vi "SubVI_Protocol_Calibration_Rev2.vi"(0 "TCP Network Connection in":refnum<k5>, 1 "ATAN scaler":dbl, 2 "Task":i32, 3 "Rest Period Length":i32, 4 "Current Level":dbl, 5 "error in (no error)":errorcluster, 6 "Total trial length":i32, 7 "Max Position":dbl, 8 "End of Imagine":i32, 9 "Target array":dbl[](array[numeric]), 10 "End of Fixate":i32, 11 "Arm Sampling Rate":u32, 17 "MidOut Proportion":dbl=0.55, 18 "Arm":string="right") -> (14 "TCP Network Connection out":refnum<k5>, 19 "error out":errorcluster)   [LabVIEW 2020]
uses:
  Global 1.vi
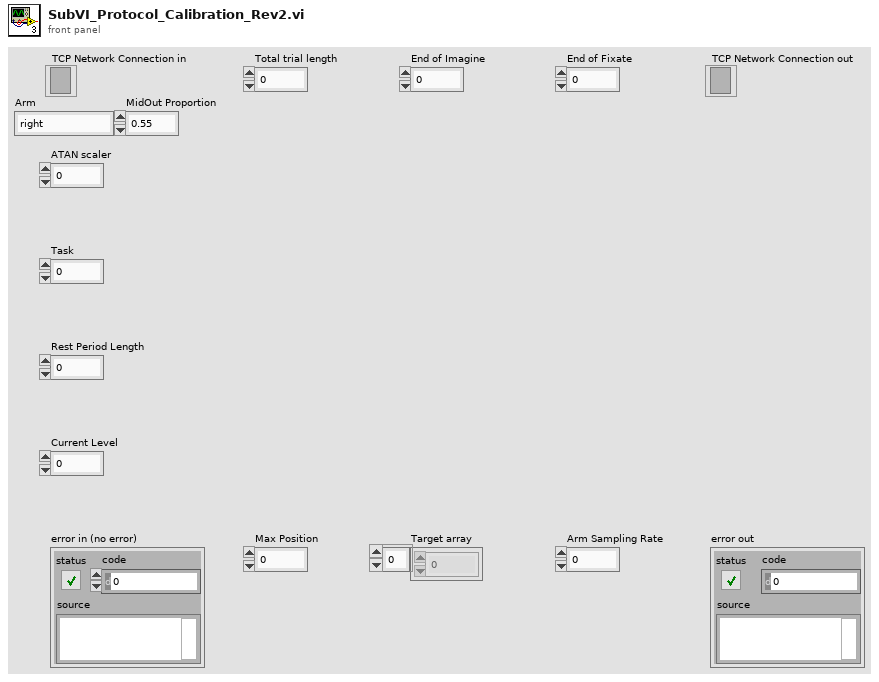
[diagram p1: front panel]
types:
  T1 = enum16{"Standard", "Buffered", "CRLF", "Immediate"}
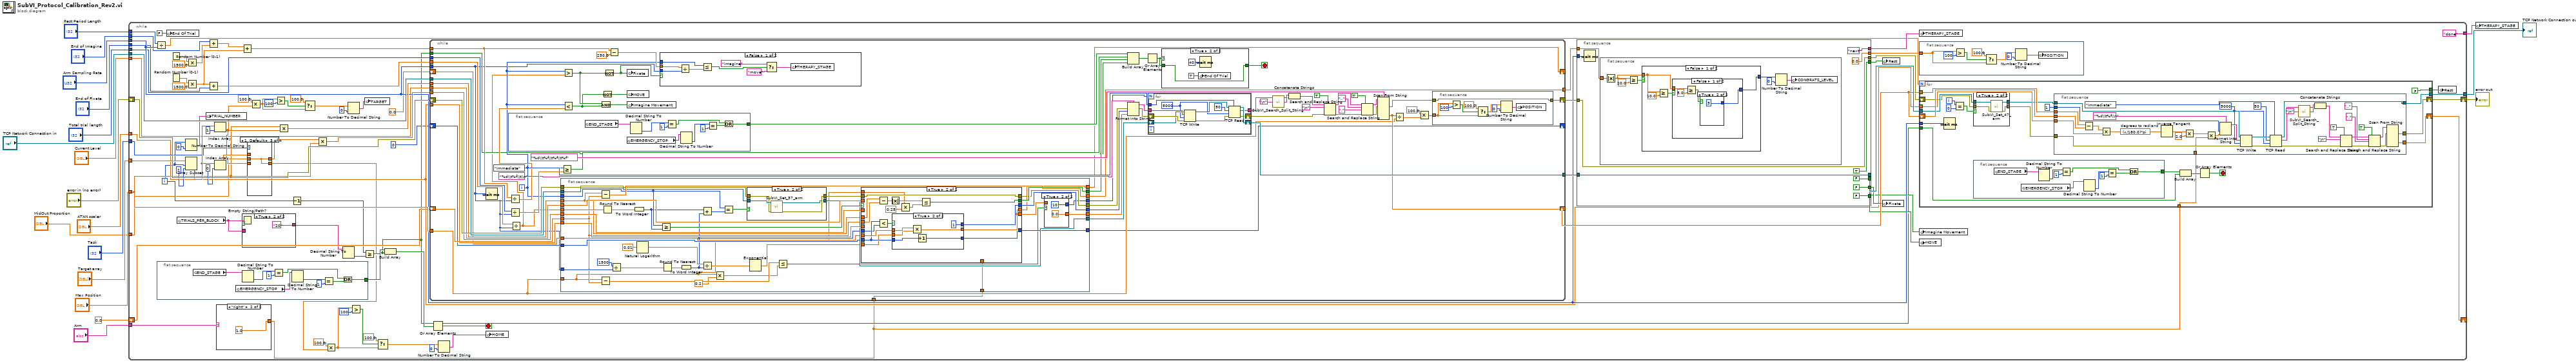
[diagram p0: block diagram]
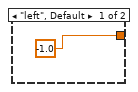
[diagram p2: hidden frame]
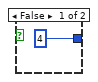
[diagram p5: hidden frame]
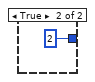
[diagram p6: hidden frame]
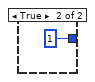
[diagram p7: hidden frame]
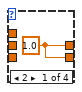
[diagram p8: hidden frame]
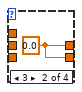
[diagram p9: hidden frame]
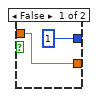
[diagram p13: hidden frame]
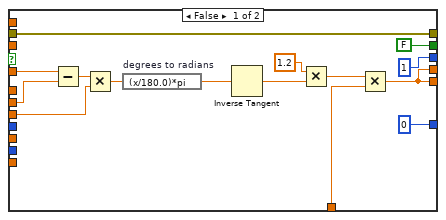
[diagram p14: hidden frame]
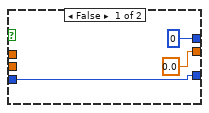
[diagram p15: hidden frame]
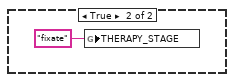
[diagram p16: hidden frame]
diagram:
  n1 = while {
    tunnel: "TCP Network Connection in" -> [w102]
    tunnel: [w64] -> w13
    shift-right: [w63] -> w14
    shift-left: "error in (no error)" -> [w101]
    tunnel: ["done" ("THERAPY_STAGE")] -> w17
    tunnel: "Arm Sampling Rate" -> [w61]
    tunnel: "Target array" -> [w99]
    tunnel: "Task" -> [w76]
    tunnel: "Max Position" -> [w71]
    tunnel: "Current Level" -> [w59]
    shift-right: [w65] -> _
    shift-left: 0.0 ("x") -> [w68]
    tunnel: "ATAN scaler" -> [w53]
    tunnel: "End of Fixate" -> [w41]
    tunnel: "End of Imagine" -> [w37]
    tunnel: "Total trial length" -> [w51]
    tunnel: "Rest Period Length" -> [w49]
    tunnel: "Arm" -> [w24]
    tunnel: "MidOut Proportion" -> [w21]
    i -> [w47]
    stop <- w29 stop-if-true
    n2 = Divide(x=w49, y=w61) -> (x/y=w60:dbl)
    n3 = flat-sequence {
      tunnel: [w105] -> w30
      frame #0 {
        n4 = global read "Global 1.vi" "END_STAGE"() -> (w113:string)
        n5 = global read "Global 1.vi" "EMERGENCY_STOP"() -> (w108:string)
        n6 = Decimal String To Number(string=w113) -> (number=w112:i32)  [unwired: 2 in, 1 out]
        n7 = Equal?(x=w112, y=1) -> (x = y?=w106:bool)
        n8 = Decimal String To Number(string=w108) -> (number=w110:i32)  [unwired: 2 in, 1 out]
        n9 = Equal?(x=w110, y=1) -> (x = y?=w107:bool)
        n10 = Or(x=w106, y=w107) -> (x .or. y?=w105:bool)
      }
    }
    n11 = global write "Global 1.vi" "End Of Trial"(FALSE ("End Of Trial")) -> ()
    n12 = Random Number (0-1)() -> (number: 0 to 1=w39:dbl)
    n13 = Random Number (0-1)() -> (number: 0 to 1=w43:dbl)
    n14 = global read "Global 1.vi" "TRIALS_PER_BLOCK"() -> (w45:string)
    n15 = Number To Decimal String(number=w47, width (-)=i16 0) -> (decimal integer string=w74:string)
    n16 = Array Subset(array=w99, index=w47, length=2) -> (w97:dbl[])
    n17 = Multiply(x=w39, y=1500.0) -> (x*y=w36:dbl)
    n18 = Multiply(x=w43, y=1500.0) -> (x*y=w34:dbl)
    n19 = global write "Global 1.vi" "TRIAL_NUMBER"(w74) -> ()
    n20 = Add(x=w37, y=w36) -> (x+y=w35:dbl)
    n21 = Add(x=w34, y=w41) -> (x+y=w40:dbl)
    n22 = Index Array(array=w97, index=1) -> (element=w79:dbl)
    n23 = Index Array(array=w97, index=0) -> (element=w94:dbl)
    n24 = case shown="\"right\"" w24 {
      tunnel: [-1.0 1.0] -> w25
      frame "left", Default {
      }
      frame "right" {
      }
    }
    n25 = Add(x=w35, y=w34) -> (x+y=w33:dbl)
    n26 = Empty String/Path?(string/path=w45) -> (empty?=w46:bool)
    n27 = case shown="True" w46 {
      tunnel: w45 -> [w114 _]
      tunnel: [w114 "20" ("TRIALS_PER_BLOCK")] -> w44
      frame False {
      }
      frame True {
      }
    }
    n28 = case shown="1, Default" w76 {
      tunnel: [w227 w228 w229 w231] -> w20
      tunnel: w94 -> [_ _ _ w231]
      tunnel: w79 -> [_ _ _ w230]
      tunnel: [w227 w228 w229 w230] -> w19
      tunnel: w21 -> [_ _ w229 _]
      frame 2 {
        w227 = 1.0
      }
      frame 3 {
        w228 = 0.0
      }
      frame 1, Default {
      }
      frame 0 {
      }
    }
    n29 = Multiply(x=100.0, y=w79) -> (x*y=w89:dbl)
    n30 = Greater?(x=w89, y=100) -> (0:w93:bool)
    n31 = Multiply(x=w71, y=w79) -> (x*y=w77:dbl)
    n32 = Decrement(x=w47) -> (x-1=w32:i32)
    n33 = Select(t=100.0, s=w93, f=w89) -> (s? t:f=w22:dbl)
    n34 = Multiply(x=w20, y=w71) -> (x*y=w78:dbl)
    n35 = Multiply(x=100.0, y=w19) -> (x*y=w83:dbl)
    n36 = Decimal String To Number(string=w44) -> (number=w48:i32)  [unwired: 2 in, 1 out]
    n37 = Number To Decimal String(number=w22, width (-)=i16 0) -> (decimal integer string=w80:string)
    n38 = Greater?(x=w83, y=100) -> (0:w87:bool)
    n39 = Greater Or Equal?(x=w32, y=w48) -> (x >= y?=w28:bool)
    n40 = global write "Global 1.vi" "TARGET"(w80) -> ()
    n41 = Select(t=100.0, s=w87, f=w83) -> (s? t:f=w23:dbl)
    n42 = Build Array(w30, w28) -> (w31:bool[])
    n43 = while {
      tunnel: [w299] -> w70
      shift-right: [w236] -> w69
      shift-left: w101 -> [w274]
      tunnel: w102 -> [w275]
      tunnel: w61 -> [w235]
      tunnel: w78 -> [w271]
      tunnel: w77 -> [w270]
      tunnel: w71 -> [w268]
      shift-right: [w276] -> w66
      shift-left: w68 -> [w272]
      tunnel: w59 -> [w273]
      tunnel: w53 -> [w259]
      tunnel: [w254] -> w52
      tunnel: w40 -> [w251]
      tunnel: w33 -> [w250]
      tunnel: w51 -> [w249]
      tunnel: w28 -> [w245]
      shift-right: [w233] -> _
      shift-left: 0.0 -> [w243]
      shift-right: [w242] -> _
      shift-left: 0 -> [w241]
      tunnel: w25 -> [w232]
      i -> [w246]
      stop <- w247 stop-if-true
      n44 = Wait (ms)(milliseconds to wait=w235) -> ()  [unwired: 1 out]
      n45 = flat-sequence {
        tunnel: [w408] -> w258
        frame #0 {
          n46 = global read "Global 1.vi" "END_STAGE"() -> (w416:string)
          n47 = global read "Global 1.vi" "EMERGENCY_STOP"() -> (w411:string)
          n48 = Decimal String To Number(string=w416) -> (number=w415:i32)  [unwired: 2 in, 1 out]
          n49 = Equal?(x=w415, y=1) -> (x = y?=w409:bool)
          n50 = Decimal String To Number(string=w411) -> (number=w413:i32)  [unwired: 2 in, 1 out]
          n51 = Equal?(x=w413, y=1) -> (x = y?=w410:bool)
          n52 = Or(x=w409, y=w410) -> (x .or. y?=w408:bool)
        }
      }
      n53 = Divide(x=w250, y=w235) -> (x/y=w269:dbl)
      n54 = Divide(x=w249, y=w235) -> (x/y=w297:dbl)
      n55 = Divide(x=w251, y=w235) -> (x/y=w244:dbl)
      n56 = flat-sequence {
        tunnel: w274 -> [w342]
        tunnel: w275 -> [w343]
        tunnel: w270 -> [w318]
        tunnel: w271 -> [w354]
        tunnel: [w346] -> w267
        tunnel: [w352] -> w265
        tunnel: [w328] -> w266
        tunnel: [w341] -> w263
        tunnel: w246 -> [w345]
        tunnel: w244 -> [w356]
        tunnel: w272 -> [w326]
        tunnel: w268 -> [w315]
        tunnel: w273 -> [w350]
        tunnel: w259 -> [w349]
        tunnel: [w348] -> w256
        tunnel: [w347] -> w254
        tunnel: [w340] -> w233
        tunnel: w243 -> [w339]
        tunnel: w241 -> [w338]
        tunnel: [w337] -> w242
        tunnel: w235 -> [w334]
        tunnel: [w327] -> w234
        tunnel: w232 -> [w319]
        frame #0 {
          n57 = Subtract(x=w318, y=w326) -> (x-y=w347:dbl)
          n58 = Subtract(x=w315, y=w326) -> (x-y=w351:dbl)
          n59 = Round To Nearest(number=w356) -> (nearest integer value=w331:dbl)
          n60 = Divide(x=1500, y=w334) -> (x/y=w333:dbl)
          n61 = To Word Integer(number=w331) -> (16bit integer=w330:i16)
          n62 = Natural Logarithm(1:0.01 ("y")) -> (0:w323:dbl)
          n63 = Greater Or Equal?(x=w345, y=w330) -> (x >= y?=w355:bool)
          n64 = Round To Nearest(number=w333) -> (nearest integer value=w332:dbl)
          n65 = To Word Integer(number=w332) -> (16bit integer=w322:i16)
          n66 = Add(x=w330, y=w322) -> (x+y=w336:i16)
          n67 = Divide(x=w323, y=w322) -> (x/y=w321:dbl)
          n68 = Multiply(x=w315, y=0.2) -> (x*y=w316:dbl)
          n69 = Equal?(x=w345, y=w336) -> (x = y?=w344:bool)
          n70 = case shown="True" w344 {
            tunnel: w343 -> [w357 w362]
            tunnel: w342 -> [w358 w361]
            tunnel: [w358 w360] -> w329
            tunnel: [w357 w359] -> w341
            frame False {
            }
            frame True {
              n71 = call "SubVI_Set_37_arm.vi"("error in (no error)"=w361, "TCP Network Connection in"=w362) -> ("error out"=w360:errorcluster, "TCP Network Connection out"=w359:refnum<k5>)  [unwired: 8 in]
            }
          }
          n72 = Exponential(1:w321) -> (0:w320:dbl)
          n73 = Less Or Equal?(x=w351, y=w316) -> (x <= y?=w325:bool)
          n74 = case shown="True" w355 {
            tunnel: w318 -> [_ w397]
            tunnel: w354 -> [w380 _]
            tunnel: w326 -> [w379 w398]
            tunnel: w350 -> [_ _]
            tunnel: [w370 w390] -> w353
            tunnel: w349 -> [w376 _]
            tunnel: [FALSE w394] -> w348
            tunnel: [1 ("input 1") w392] -> w346
            tunnel: [w370 w390] -> w340
            tunnel: w339 -> [_ w391]
            tunnel: w338 -> [_ w388]
            tunnel: [0 w389] -> w337
            tunnel: w322 -> [_ w387]
            tunnel: w329 -> [w368 w386]
            tunnel: [w368 w386] -> w328
            tunnel: w320 -> [_ w385]
            tunnel: w319 -> [w367 _]
            tunnel: w315 -> [_ w383]
            frame False {
              n75 = Subtract(x=w380, y=w379) -> (x-y=w378:dbl)
              n76 = Multiply(x=w378, y=w376) -> (x*y=w377:dbl)
              n77 = expression code="(x/180.0)*pi" "degrees to radians"(w377) -> (w381:dbl)
              n78 = Inverse Tangent(1:w381) -> (0:w375:dbl)
              n79 = Multiply(x=1.2, y=w375) -> (x*y=w373:dbl)
              n80 = Multiply(x=w373, y=w367) -> (x*y=w370:dbl)
            }
            frame True {
              n81 = Subtract(x=w397, y=w398) -> (x-y=w396:dbl)
              n82 = Less?(x=w388, y=w387) -> (x < y?=w393:bool)
              n83 = Absolute Value(x=w396) -> (abs(x)=w395:dbl)
              n84 = case shown="True" w393 {
                tunnel: [0 ("input 1") 1 ("input 1")] -> w392
                tunnel: [0.0 w405] -> w390
                tunnel: w391 -> [_ w406]
                tunnel: w388 -> [w399 w404]
                tunnel: [w399 w403] -> w389
                tunnel: w385 -> [_ w402]
                frame False {
                }
                frame True {
                  n85 = Multiply(x=w406, y=w402) -> (x*y=w405:dbl)
                  n86 = Increment(x=w404) -> (x+1=w403:i32)
                }
              }
              n87 = Multiply(x=w383, y=0.25) -> (x*y=w382:dbl)
              n88 = Less Or Equal?(x=w395, y=w382) -> (x <= y?=w394:bool)
            }
          }
          n89 = case shown="True" w325 {
            tunnel: w353 -> [w364 _]
            tunnel: [w364 0.0] -> w352
            tunnel: [1 10] -> w327
            frame False {
            }
            frame True {
            }
          }
        }
      }
      n90 = Greater Or Equal?(x=w246, y=w297) -> (x >= y?=w257:bool)
      n91 = Greater?(x=w246, y=w244) -> (0:w296:bool)
      n92 = Less?(x=w246, y=w269) -> (x < y?=w295:bool)
      n93 = And(x=w296, y=w295) -> (x .and. y?=w261:bool)
      n94 = Not(x=w295) -> (.not. x?=w260:bool)
      n95 = Not(x=w296) -> (.not. x?=w262:bool)
      n96 = Subtract(x=w250, y=250.0) -> (x-y=w253:dbl)
      n97 = global write "Global 1.vi" "Fixate"(w262) -> ()
      n98 = global write "Global 1.vi" "MOVE"(w260) -> ()
      n99 = global write "Global 1.vi" "Imagine Movement"(w261) -> ()
      n100 = case shown="False" w262 {
        tunnel: w246 -> [w432 _]
        tunnel: w235 -> [w427 _]
        tunnel: w253 -> [w425 _]
        frame False {
          n101 = Divide(x=w425, y=w427) -> (x/y=w428:dbl)
          n102 = Less Or Equal?(x=w432, y=w428) -> (x <= y?=w431:bool)
          n103 = Select(t="imagine" ("THERAPY_STAGE"), s=w431, f="move" ("THERAPY_STAGE")) -> (s? t:f=w426:string)
          n104 = global write "Global 1.vi" "THERAPY_STAGE"(w426) -> ()
        }
        frame True {
          n105 = global write "Global 1.vi" "THERAPY_STAGE"("fixate" ("THERAPY_STAGE")) -> ()
        }
      }
      n106 = Build Array(w258, w257, w256, w245) -> (w255:bool[])
      n107 = Format Into String(format string="%d\\t%f\\t\\n", error in=w266, w267, w265) -> (resulting string=w280:string, error out=w264:errorcluster)  [unwired: 1 in]
      n108 = Or Array Elements(Boolean array=w255) -> (logical OR=w248:bool)
      n109 = for {
        N: w234 -> [_]
        tunnel: T1."Immediate" ("mode (standard)") -> [w308]
        tunnel: [w305] -> w292
        tunnel: w280 -> [w304]
        shift-right: [w301] -> w240
        shift-left: w264 -> [w303]
        shift-right: [w310] -> w299
        shift-left: w263 -> [w302]
        w300 = 5000 ("timeout ms (25000)")
        n110 = TCP Write(connection ID=w302, data in=w304, error in (no error)=w303, 9:w300) -> (connection ID out=w307:refnum<k5>, error out=w306:errorcluster)  [unwired: 1 out]
        n111 = TCP Read(connection ID=w307, bytes to read=50, error in (no error)=w306, 7:w308, 9:w300) -> (connection ID out=w310:refnum<k5>, data out=w305:string, error out=w301:errorcluster)
      }
      n112 = case shown="True" w248 {
        tunnel: w248 -> [w311 w314]
        tunnel: [w311 w314] -> w247
        frame False {
        }
        frame True {
          n113 = global write "Global 1.vi" "End Of Trial"(TRUE ("End Of Trial")) -> ()
          n114 = Wait (ms)(milliseconds to wait=u32 40) -> ()  [unwired: 1 out]
        }
      }
      n115 = call <userlib>:"SubVI_Search_Split_String.vi"("search string/char (-)"="\n", "string"=w292) -> ("substring after match"=w290:string, "substring before match"=w279:string)  [unwired: 1 in, 1 out]
      n116 = Concatenate Strings(w290, w279) -> (w287:string)
      n117 = Search and Replace String(replace all?=TRUE ("replace all? (F)"), input string=w287, search string="\n", error in=w240) -> (result string=w282:string, error out=w239:errorcluster)  [unwired: 4 in, 2 out]
      n118 = Search and Replace String(replace all?=TRUE ("replace all? (F)"), input string=w282, search string="..", replace string="." ("replace string (\"\")"), error in=w239) -> (result string=w278:string, error out=w238:errorcluster)  [unwired: 3 in, 2 out]
      n119 = Scan From String(format string="%d\\t%f\\t%f\\t%f", input string=w278, error in=w238) -> (error out=w237:errorcluster, output 3=w276:dbl)  [unwired: 8 in, 2 out]
      n120 = Divide(x=w276, y=w268) -> (x/y=w294:dbl)
      n121 = Multiply(x=100.0, y=w294) -> (x*y=w277:dbl)
      n122 = flat-sequence {
        tunnel: w277 -> [w418]
        tunnel: w237 -> [w417]
        tunnel: [w417] -> w236
        frame #0 {
          n123 = Greater?(x=w418, y=100) -> (0:w423:bool)
          n124 = Select(t=100.0, s=w423, f=w418) -> (s? t:f=w420:dbl)
          n125 = Number To Decimal String(number=w420, width (-)=i16 0) -> (decimal integer string=w419:string)
          n126 = global write "Global 1.vi" "POSITION"(w419) -> ()
        }
      }
    }
    n127 = Or Array Elements(Boolean array=w31) -> (logical OR=w29:bool)
    n128 = Number To Decimal String(number=w23, width (-)=i16 0) -> (decimal integer string=w81:string)
    n129 = global write "Global 1.vi" "HOME"(w81) -> ()
    n130 = flat-sequence {
      tunnel: [FALSE ("MOVE")] -> w56
      tunnel: [FALSE ("Imagine Movement")] -> w57
      tunnel: [TRUE ("Rest")] -> w55
      tunnel: [FALSE ("Fixate")] -> w58
      tunnel: w61 -> [w196]
      tunnel: ["next" ("THERAPY_STAGE")] -> w73
      tunnel: [0.0 ("Arm_position")] -> w72
      tunnel: [w193] -> w67
      tunnel: w70 -> [w193]
      tunnel: [w192] -> w62
      tunnel: w69 -> [w192]
      tunnel: w52 -> [w191]
      frame #0 {
        n131 = Wait (ms)(milliseconds to wait=w196) -> ()  [unwired: 1 out]
        n132 = flat-sequence {
          tunnel: w191 -> [w202]
          frame #0 {
            n133 = Absolute Value(x=w202) -> (abs(x)=w201:dbl)
            n134 = Greater Or Equal?(x=w201, y=20.0) -> (x >= y?=w206:bool)
            n135 = case shown="False" w206 {
              tunnel: [w209 1] -> w204
              tunnel: w201 -> [w208 _]
              frame False {
                n136 = Greater Or Equal?(x=w208, y=10.0) -> (x >= y?=w211:bool)
                n137 = case shown="False" w211 {
                  tunnel: [w213 2] -> w209
                  tunnel: w208 -> [w215 _]
                  frame False {
                    n138 = Greater Or Equal?(x=w215, y=5.0) -> (x >= y?=w212:bool)
                    n139 = case shown="True" w212 {
                      tunnel: [4 3] -> w213
                      frame False {
                      }
                      frame True {
                      }
                    }
                  }
                  frame True {
                  }
                }
              }
              frame True {
              }
            }
            n140 = Number To Decimal String(number=w204, width (-)=i16 0) -> (decimal integer string=w203:string)
            n141 = global write "Global 1.vi" "CONGRATS_LEVEL"(w203) -> ()
          }
        }
      }
    }
    n142 = global write "Global 1.vi" "Rest"(w55) -> ()
    n143 = global write "Global 1.vi" "Fixate"(w58) -> ()
    n144 = global write "Global 1.vi" "THERAPY_STAGE"(w73) -> ()
    n145 = flat-sequence {
      tunnel: w72 -> [w220]
      frame #0 {
        n146 = Greater?(x=w220, y=100) -> (0:w225:bool)
        n147 = Select(t=100.0, s=w225, f=w220) -> (s? t:f=w222:dbl)
        n148 = Number To Decimal String(number=w222, width (-)=i16 0) -> (decimal integer string=w221:string)
        n149 = global write "Global 1.vi" "POSITION"(w221) -> ()
      }
    }
    n150 = for {
      N: w60 -> [_]
      shift-right: [w133] -> w63
      shift-left: w62 -> [w126]
      tunnel: [FALSE ("Rest")] -> w54
      tunnel: w67 -> [w127]
      tunnel: w61 -> [w135]
      tunnel: [w132] -> w64
      shift-right: [w131] -> w65
      shift-left: w66 -> [w129]
      tunnel: w66 -> [w130]
      tunnel: w53 -> [w128]
      tunnel: w28 -> [w119]
      tunnel: w25 -> [w116]
      i -> [w122]
      stop <- w117 stop-if-true
      n151 = Wait (ms)(milliseconds to wait=w135) -> ()  [unwired: 1 out]
      n152 = Equal?(x=w122, y=0) -> (x = y?=w121:bool)
      n153 = case shown="True" w121 {
        tunnel: w127 -> [w137 w142]
        tunnel: w126 -> [w138 w141]
        tunnel: [w138 w140] -> w124
        tunnel: [w137 w139] -> w125
        frame False {
        }
        frame True {
          n154 = call "SubVI_Set_47_arm.vi"("error in (no error)"=w141, "TCP Network Connection in"=w142) -> ("error out"=w140:errorcluster, "TCP Network Connection out"=w139:refnum<k5>)  [unwired: 8 in]
        }
      }
      n155 = flat-sequence {
        tunnel: [w143] -> w118
        frame #0 {
          n156 = global read "Global 1.vi" "END_STAGE"() -> (w151:string)
          n157 = global read "Global 1.vi" "EMERGENCY_STOP"() -> (w146:string)
          n158 = Decimal String To Number(string=w151) -> (number=w150:i32)  [unwired: 2 in, 1 out]
          n159 = Equal?(x=w150, y=1) -> (x = y?=w144:bool)
          n160 = Decimal String To Number(string=w146) -> (number=w148:i32)  [unwired: 2 in, 1 out]
          n161 = Equal?(x=w148, y=1) -> (x = y?=w145:bool)
          n162 = Or(x=w144, y=w145) -> (x .or. y?=w143:bool)
        }
      }
      n163 = flat-sequence {
        tunnel: 1 ("input 1") -> [w184]
        tunnel: [w183] -> w132
        tunnel: [w154] -> w133
        tunnel: w125 -> [w182]
        tunnel: w124 -> [w181]
        tunnel: [w170] -> w131
        tunnel: w130 -> [w167]
        tunnel: w129 -> [w166]
        tunnel: w128 -> [w161]
        tunnel: w116 -> [w152]
        frame #0 {
          w153 = 5000 ("timeout ms (25000)")
          n164 = Subtract(x=w167, y=w166) -> (x-y=w163:dbl)
          n165 = Multiply(x=w163, y=w161) -> (x*y=w162:dbl)
          n166 = expression code="(x/180.0)*pi" "degrees to radians"(w162) -> (w164:dbl)
          n167 = Inverse Tangent(1:w164) -> (0:w160:dbl)
          n168 = Multiply(x=w160, y=2.0) -> (x*y=w159:dbl)
          n169 = Multiply(x=w159, y=w152) -> (x*y=w165:dbl)
          n170 = Format Into String(format string="%d\\t%f\\n", w184, w165) -> (resulting string=w185:string)  [unwired: 2 in, 1 out]
          n171 = TCP Write(connection ID=w182, data in=w185, error in (no error)=w181, 9:w153) -> (connection ID out=w188:refnum<k5>, error out=w187:errorcluster)  [unwired: 1 out]
          n172 = TCP Read(connection ID=w188, bytes to read=50, error in (no error)=w187, 7:T1."Immediate" ("mode (standard)"), 9:w153) -> (connection ID out=w183:refnum<k5>, data out=w171:string, error out=w157:errorcluster)
          n173 = call <userlib>:"SubVI_Search_Split_String.vi"("search string/char (-)"="\n", "string"=w171) -> ("substring after match"=w179:string, "substring before match"=w173:string)  [unwired: 1 in, 1 out]
          n174 = Concatenate Strings(w179, w173) -> (w177:string)
          n175 = Search and Replace String(replace all?=TRUE ("replace all? (F)"), input string=w177, search string="\n", error in=w157) -> (result string=w174:string, error out=w156:errorcluster)  [unwired: 4 in, 2 out]
          n176 = Search and Replace String(replace all?=TRUE ("replace all? (F)"), input string=w174, search string="..", replace string="." ("replace string (\"\")"), error in=w156) -> (result string=w172:string, error out=w155:errorcluster)  [unwired: 3 in, 2 out]
          n177 = Scan From String(input string=w172, error in=w155) -> (error out=w154:errorcluster, output 3=w170:dbl)  [unwired: 9 in, 2 out]
        }
      }
      n178 = Build Array(w118, w119) -> (w120:bool[])
      n179 = Or Array Elements(Boolean array=w120) -> (logical OR=w117:bool)
    }
    n180 = global write "Global 1.vi" "Imagine Movement"(w57) -> ()
    n181 = global write "Global 1.vi" "MOVE"(w56) -> ()
    n182 = global write "Global 1.vi" "Rest"(w54) -> ()
  }
  "error out" <- w14
  "TCP Network Connection out" <- w13
  n183 = global write "Global 1.vi" "THERAPY_STAGE"(w17) -> ()
